vi "Echo_Record_Values.vi"(10 "Data":dbl[](array[numeric]), 11 "Record":bool) -> (3 "Out":dbl[][](graph))   [LabVIEW 2012]
panel:
  # "This VI is contained within Echo Record\n\nIt does not need to be placed anywhere.\n\nIt takes inputs (fed to it by Echo Record)\nand tacks them on to the end of an array\n\nUpon being told to stop recording, it\nresets the array and outputs the data\n(which will be converted to a standard\nsize (250 x 11)  and written to a\nspreadsheet by Echo Record)"
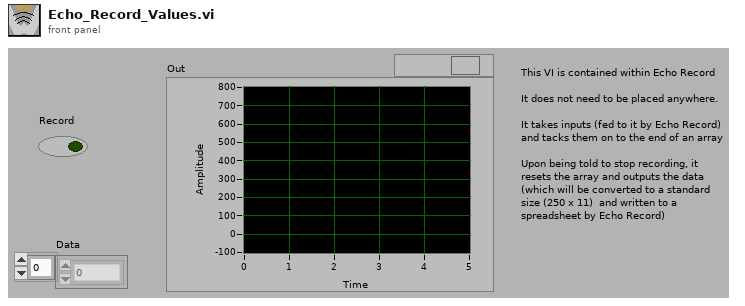
[diagram p1: front panel]
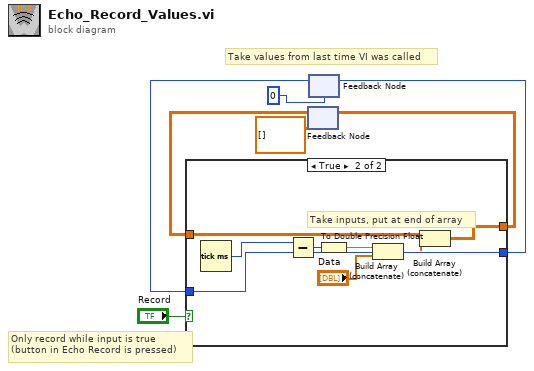
[diagram p0: block diagram]
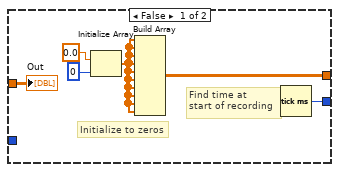
[diagram p2: hidden frame]
diagram:
  # "Take values from last time VI was called"
  # "Only record while input is true\n(button in Echo Record is pressed)"
  n1 = feedback #1(dbl[][] []) -> (w7:dbl[][])
  n2 = feedback #2(u32 0 ("millisecond timer value")) -> (w3:u32)
  n3 = case shown="True" "Record" {
    tunnel: w3 -> [_ w16]
    tunnel: w7 -> [w9 w18]
    tunnel: [w11 w17] -> w5
    tunnel: [w10 w16] -> w4
    frame False {
      # "Find time at\nstart of recording"
      # "Initialize to zeros"
      n4 = Initialize Array(0.0 ("element"), 0 ("dimension size")) -> (w8:dbl[])
      n5 = Build Array(w8, w8, w8, w8, w8, w8, w8, w8, w8, w8) -> (w11:dbl[][])
      n6 = Tick Count (ms)() -> (millisecond timer value=w10:u32)
      "Out" <- w9
    }
    frame True {
      # "Take inputs, put at end of array"
      n7 = Tick Count (ms)() -> (millisecond timer value=w21:u32)
      n8 = Subtract(x=w21, y=w16) -> (x-y=w20:u32)
      n9 = To Double Precision Float(number=w20) -> (double precision float=w19:dbl)
      n10 = Build Array (concatenate)(w19, "Data") -> (w14:dbl[])
      n11 = Build Array (concatenate)(w18, w14) -> (w17:dbl[][])
    }
  }
  n12 = feedback-in #1(w5) -> ()
  n13 = feedback-in #2(w4) -> ()
